vi "SP Save Formatting with Test Run.vi"(7 "Display":T1={"Lock Control"=FALSE, "Retain Settings"=TRUE, "Formatted Data"=FALSE, "Plot Orientation"=enum."Single", "Plot Controls"=[{"Trace Orientation"=enum."Overlay", "Frequency"={"Change Frequency"=FALSE, "Start"=500.0, "Stop"=1500.0, "Units"=enum."MHz"}, "Markers"=[], "Traces"=[]}, {"Trace Orientation"=enum."Overlay", "Frequency"={"Change Frequency"=FALSE, "Start"=500.0, "Stop"=1500.0, "Units"=enum."MHz"}, "Markers"=[], "Traces"=[]}, {"Trace Orientation"=enum."Overlay", "Frequency"={"Change Frequency"=FALSE, "Start"=500.0, "Stop"=1500.0, "Units"=enum."MHz"}, "Markers"=[], "Traces"=[]}, {"Trace Orientation"=enum."Overlay", "Frequency"={"Change Frequency"=FALSE, "Start"=500.0, "Stop"=1500.0, "Units"=enum."MHz"}, "Markers"=[], "Traces"=[]}]} {"Plot Controls"."Traces"."Reference" format="%#.2g"; "Plot Controls"."Traces"."Display Data" items=["Data", "Memory", "Data/Memory"]; "Plot Controls"."Traces"."Format" items=["Log Mag", "Phase", "Expanded Phase", "Delay", "Smith", "Polar", "Lin Mag", "SWR", "Loss", "Real", "Imaginary"]; "Plot Controls"."Traces"."Scale" min=0.001 step=1.0 format="%#.2g"; "Plot Controls"."Traces"."Position" min=0.0 max=10.0; "Plot Controls"."Frequency"."Stop" format="%.3g"; "Plot Controls"."Frequency"."Start" format="%.3g"}, 8 "error in (no error)":errorcluster, 9 "Channel Name In (Display Settings)":string="Display Settings", 10 "Group Name In":string, 11 "TDMS File Ref In":refnum<k34>) -> (0 "error out":errorcluster, 1 "Channel Name Out":string, 2 "Group Name Out":string, 3 "TDMS File Ref Out":refnum<k34>)   [LabVIEW 2011]
uses:
  TypeDefs/SP Display Parameters.ctl
  TypeDefs/SP Display Plot Controls Cluster.ctl
  TypeDefs/SP Frequency Units.ctl
  TypeDefs/SP Marker Cluster.ctl
  TypeDefs/SP Marker Type.ctl
  TypeDefs/SP Display Trace Controls.ctl
  TypeDefs/SP Display Format.ctl
  TypeDefs/SP Display Data.ctl
panel:
  # "Div"
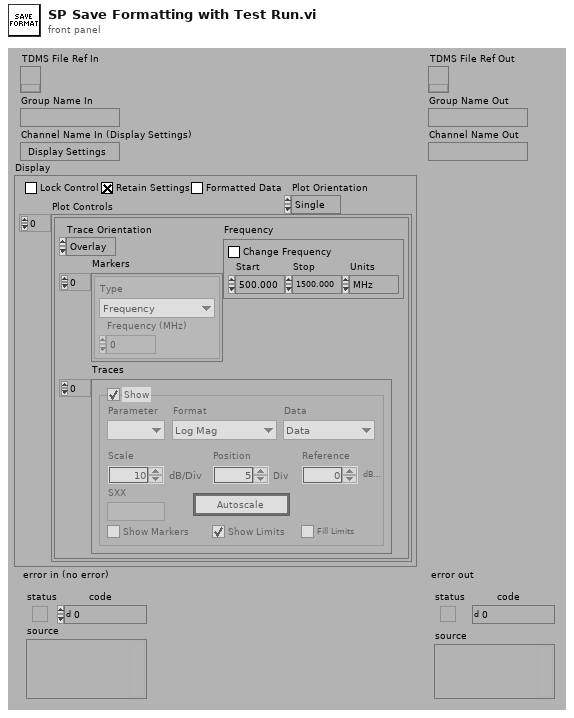
[diagram p1: front panel]
types:
  T1 = typedef "SP Display Parameters.ctl" = cluster{"Lock Control":bool, "Retain Settings":bool, "Formatted Data":bool, "Plot Orientation":enum32{"Single", "Dual", "Quad"}, "Plot Controls":T2[]}
  T2 = typedef "SP Display Plot Controls Cluster.ctl" = cluster{"Trace Orientation":enum32{"Overlay", "Split"}, "Frequency":cluster{"Change Frequency":bool, "Start":dbl, "Stop":dbl, "Units":T3}, "Markers":T4[], "Traces":T6[]}
  T3 = typedef "SP Frequency Units.ctl" = enum16{"Hz", "kHz", "MHz", "GHz", "Points"}
  T4 = typedef "SP Marker Cluster.ctl" = cluster{"Type":T5, "Frequency (MHz)":dbl}
  T5 = typedef "SP Marker Type.ctl" = enum16{"Frequency", "Trace Maximum", "Trace Minimum", "Limit Maximum", "Limit Minimum"}
  T6 = typedef "SP Display Trace Controls.ctl" = cluster{"Trace On":bool, "Measure":i32, "Format":T7, "Autoscale":bool, "Reference":dbl, "\nRefUnit":string, "Position":dbl, "Scale":dbl, "ScaleUnit":string, "LimitOn":bool, "LimitFill":bool, "Display Data":T8, "Show Markers":bool, "SXX":string}
  T7 = typedef "SP Display Format.ctl" = i32
  T8 = typedef "SP Display Data.ctl" = u16
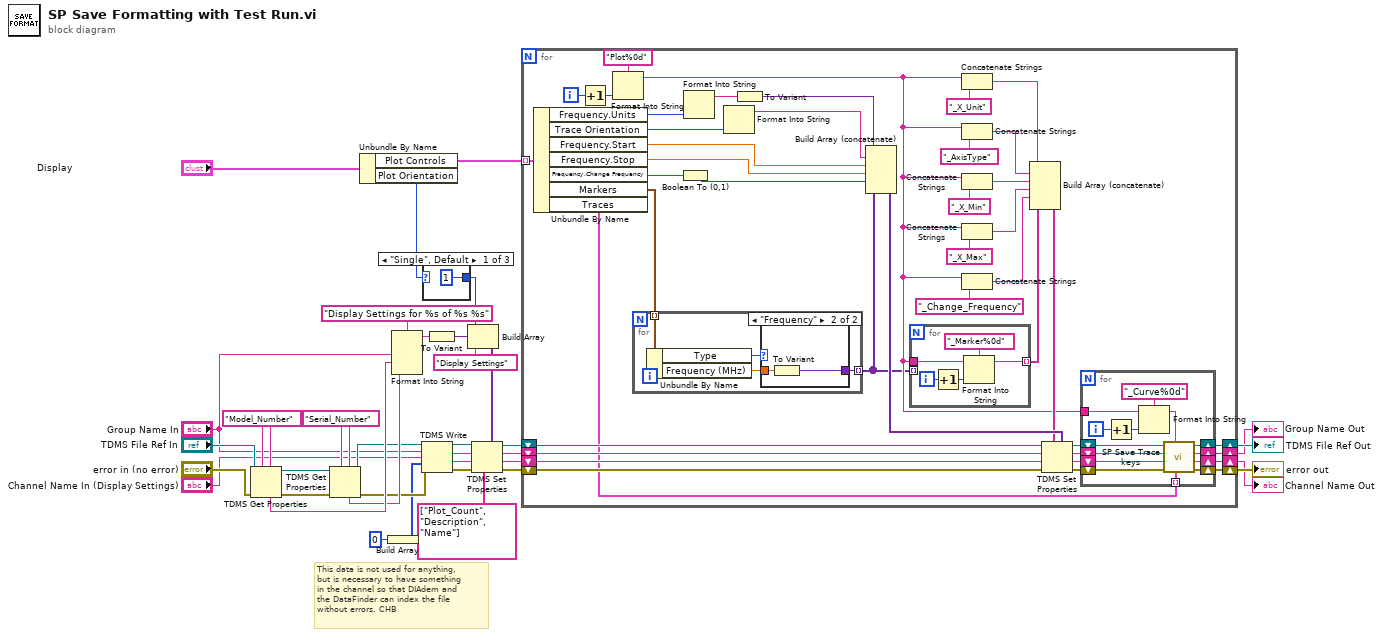
[diagram p0: block diagram]
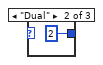
[diagram p2: hidden frame]
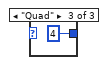
[diagram p3: hidden frame]
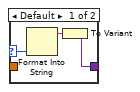
[diagram p4: hidden frame]
diagram:
  w21 = "Serial_Number" ("sxFieldId")
  w20 = "Model_Number" ("sxFieldId")
  # "This data is not used for anything,\nbut is necessary to have something\nin the channel so that DIAdem and\nthe DataFinder can index the file\nwithout errors. CHB"
  n1 = TDMS Get Properties(5:w20, 7:w20, 8:"error in (no error)", 11:"TDMS File Ref In") -> (0:w23:errorcluster, 3:w22:refnum<k34>, 4:w18:string)  [unwired: 5 out]
  n2 = TDMS Get Properties(5:w21, 7:w21, 8:w23, 11:w22) -> (0:w9:errorcluster, 3:w10:refnum<k34>, 4:w17:string)  [unwired: 5 out]
  n3 = Unbundle By Name("Display") -> ("Plot Controls"=w35:T2[], "Plot Orientation"=w11:enum32{"Single", "Dual", "Quad"})
  n4 = Build Array(0 ("sxFieldId")) -> (w1:i32[])
  n5 = Format Into String(format string="Display Settings for %s of %s %s" ("sxFieldId"), "Group Name In", w18, w17) -> (resulting string=w16:string)  [unwired: 2 in, 1 out]
  n6 = TDMS Write(0:w10, 5:"Group Name In", 7:"Channel Name In (Display Settings)", 9:w1, 11:w9) -> (4:w7:refnum<k34>, 6:w4:string, 8:w3:string, 15:w8:errorcluster)  [unwired: 1 in]
  n7 = case shown="\"Single\", Default" w11 {
    tunnel: [1 ("sxFieldId") 2 ("sxFieldId") 4 ("sxFieldId")] -> w15
    frame "Single", Default {
    }
    frame "Dual" {
    }
    frame "Quad" {
    }
  }
  n8 = To Variant(anything=w16) -> (Variant=w14:variant)
  n9 = Build Array(w15, w14, "Display Settings" ("sxFieldId")) -> (w12:variant[])
  n10 = TDMS Set Properties(5:w12, 7:string[] ["Plot_Count", "Description", "Name"], 8:w8, 9:w3, 10:w4, 11:w7) -> (0:w29:errorcluster, 1:w31:string, 2:w32:string, 3:w30:refnum<k34>)
  n11 = for {
    tunnel: w35 -> [w81] mode=indexing
    shift-right: [w55] -> w34
    shift-left: w29 -> [w72]
    shift-right: [w57] -> w33
    shift-left: w30 -> [w71]
    shift-right: [w50] -> w28
    shift-left: w32 -> [w70]
    shift-right: [w49] -> w27
    shift-left: w31 -> [w53]
    i -> [w79]
    n12 = Unbundle By Name(w81) -> ("Frequency.Units"=w77:T3, "Trace Orientation"=w62:enum32{"Overlay", "Split"}, "Frequency.Start"=w43:dbl, "Frequency.Stop"=w42:dbl, "Frequency.Change Frequency"=w48:bool, "Markers"=w41:T4[], "Traces"=w52:T6[])
    n13 = Increment(x=w79) -> (x+1=w73:i32)
    n14 = Format Into String(format string="Plot%0d" ("sxFieldId"), w73) -> (resulting string=w45:string)  [unwired: 2 in, 1 out]
    n15 = for {
      tunnel: w41 -> [w85] mode=indexing
      tunnel: [w82] -> w40 mode=indexing
      n16 = Unbundle By Name(w85) -> ("Type"=w84:T5, "Frequency (MHz)"=w83:dbl)
      n17 = case shown="\"Frequency\"" w84 {
        selector: w84 -> [w88 _]
        tunnel: w83 -> [_ w90]
        tunnel: [w86 w89] -> w82
        frame Default {
          n18 = Format Into String(w88) -> (resulting string=w87:string)  [unwired: 3 in, 1 out]
          n19 = To Variant(anything=w87) -> (Variant=w86:variant)
        }
        frame "Frequency" {
          n20 = To Variant(anything=w90) -> (Variant=w89:variant)
        }
      }
    }
    n21 = Boolean To (0,1)(Boolean=w48) -> (0, 1=w47:i16)
    n22 = Format Into String(w77) -> (resulting string=w64:string)  [unwired: 3 in, 1 out]
    n23 = Format Into String(w62) -> (resulting string=w61:string)  [unwired: 3 in, 1 out]
    n24 = To Variant(anything=w64) -> (Variant=w63:variant)
    n25 = Build Array (concatenate)(w63, w61, w43, w42, w47, w40) -> (w60:variant[])
    n26 = for {
      tunnel: [w106] -> w65 mode=indexing
      tunnel: w40 -> [_] mode=indexing
      tunnel: w45 -> [w105]
      i -> [w108]
      n27 = Increment(x=w108) -> (x+1=w107:i32)
      n28 = Format Into String(format string="_Marker%0d" ("sxFieldId"), initial string=w105, w107) -> (resulting string=w106:string)  [unwired: 1 in, 1 out]
    }
    n29 = Concatenate Strings(w45, "_X_Unit" ("sxFieldId")) -> (w68:string)
    n30 = Concatenate Strings(w45, "_AxisType" ("sxFieldId")) -> (w67:string)
    n31 = Concatenate Strings(w45, "_X_Min" ("sxFieldId")) -> (w69:string)
    n32 = Concatenate Strings(w45, "_X_Max" ("sxFieldId")) -> (w66:string)
    n33 = Concatenate Strings(w45, "_Change_Frequency" ("sxFieldId")) -> (w44:string)
    n34 = Build Array (concatenate)(w68, w67, w69, w66, w44, w65) -> (w59:string[])
    n35 = TDMS Set Properties(5:w60, 7:w59, 8:w72, 9:w53, 10:w70, 11:w71) -> (0:w56:errorcluster, 1:w51:string, 2:w54:string, 3:w58:refnum<k34>)
    n36 = for {
      shift-right: [w99] -> w57
      shift-left: w58 -> [w100]
      shift-right: [w97] -> w55
      shift-left: w56 -> [w98]
      tunnel: w52 -> [w95] mode=indexing
      shift-right: [w93] -> w50
      shift-left: w54 -> [w96]
      shift-right: [w92] -> w49
      shift-left: w51 -> [w94]
      tunnel: w45 -> [w91]
      i -> [w103]
      n37 = Increment(x=w103) -> (x+1=w102:i32)
      n38 = Format Into String(format string="_Curve%0d" ("sxFieldId"), initial string=w91, w102) -> (resulting string=w101:string)  [unwired: 1 in, 1 out]
      n39 = call "SP Save Trace keys.vi"("Trace"=w95, "Prefix"=w101, "error in (no error)"=w98, "Channel Name In"=w94, "Group Name In"=w96, "TDMS File Ref In"=w100) -> ("error out"=w97:errorcluster, "Channel Name Out"=w92:string, "Group Name Out"=w93:string, "TDMS File Ref Out"=w99:refnum<k34>)  [unwired: 2 out]
    }
  }
  "error out" <- w34
  "TDMS File Ref Out" <- w33
  "Group Name Out" <- w28
  "Channel Name Out" <- w27
